vi "terminal_length_integrated.vi"(0 "ROI Ref":T3 {"Contours"."Type" items=["No Selection", "Point", "Line", "Rectangle", "Oval", "Polygon", "Free", "Annulus", "Unused2", "Unused3", "Broken Line", "Free Hand Line", "Rotated Rectangle"]}, 1 "Edge Options ROI Ref":T6={"Edge Polarity"=2, "Kernel Size"=5, "Width"=5, "Minimum Edge Strength"=50.0, "Interpolation Type"=enum."Zero Order", "Data Processing Method"=enum."Average"} {"Edge Polarity" items=["All Edges", "Rising Edges", "Falling Edges"]; "Minimum Edge Strength" format="%.2f"; "Width" step=2; "Kernel Size" step=2}, 2 "Search Direction ROI Ref":u32(ring)=3 items=["Left to Right", "Right to Left", "Top to Bottom", "Bottom to Top"], 3 "Line Options ROI Ref":T4={"Number of Lines"=1, "Type"=enum."First Edge Rake", "Min. Score"=10.0, "Max. Score"=1000.0, "Orientation"=0.0, "Angle Range"=30.0, "Angle Tolerance"=1.0, "Step Size"=5, "Min. SNR (db)"=0.0, "Min. Points (%)"=25.0, "Hough Iterations"=5} {"Min. Points (%)" min=0.0 max=100.0; "Min. SNR (db)" min=0.0; "Max. Score" min=0.0 max=1024.0; "Min. Score" min=0.0 max=1024.0 step=1.0}, 4 "ROI 1":T3 {"Contours"."Type" items=["No Selection", "Point", "Line", "Rectangle", "Oval", "Polygon", "Free", "Annulus", "Unused2", "Unused3", "Broken Line", "Free Hand Line", "Rotated Rectangle"]}, 5 "Edge Options ROI 1":T6={"Edge Polarity"=2, "Kernel Size"=5, "Width"=5, "Minimum Edge Strength"=50.0, "Interpolation Type"=enum."Zero Order", "Data Processing Method"=enum."Average"} {"Edge Polarity" items=["All Edges", "Rising Edges", "Falling Edges"]; "Minimum Edge Strength" format="%.2f"; "Width" step=2; "Kernel Size" step=2}, 6 "Search Direction ROI 1":u32(ring)=1 items=["Left to Right", "Right to Left", "Top to Bottom", "Bottom to Top"], 7 "error in (no error)":errorcluster, 8 "Image In":T8(plugin-control), 9 "Line Options ROI 1":T4={"Number of Lines"=1, "Type"=enum."First Edge Rake", "Min. Score"=10.0, "Max. Score"=1000.0, "Orientation"=0.0, "Angle Range"=30.0, "Angle Tolerance"=1.0, "Step Size"=5, "Min. SNR (db)"=0.0, "Min. Points (%)"=25.0, "Hough Iterations"=5} {"Min. Points (%)" min=0.0 max=100.0; "Min. SNR (db)" min=0.0; "Max. Score" min=0.0 max=1024.0; "Min. Score" min=0.0 max=1024.0 step=1.0}, 10 "Calibrated Image":T8, 11 "Edge Options ROI 2":T6={"Edge Polarity"=2, "Kernel Size"=5, "Width"=5, "Minimum Edge Strength"=50.0, "Interpolation Type"=enum."Zero Order", "Data Processing Method"=enum."Average"} {"Edge Polarity" items=["All Edges", "Rising Edges", "Falling Edges"]; "Minimum Edge Strength" format="%.2f"; "Width" step=2; "Kernel Size" step=2}, 12 "ROI 2":T3 {"Contours"."Type" items=["No Selection", "Point", "Line", "Rectangle", "Oval", "Polygon", "Free", "Annulus", "Unused2", "Unused3", "Broken Line", "Free Hand Line", "Rotated Rectangle"]}, 13 "Scan Direction ROI 2":u16(ring) items=["Left To Right", "Right To Left", "Top To Bottom", "Bottom To Top"], 14 "Process ROI 2":T2(ring), 15 "Step Size ROI 2":u32=5) -> (19 "overlay arrow lines":T1, 20 "Terminal Length":sgl, 27 "error out":errorcluster)   [LabVIEW 2019, in "Algorithm.lvclass"]
uses:
  FrameworkOverrides/Algorithm.lvclass
  <vilib>/vision/NI_Vision_Development_Module.lvlib
  <vilib>/vision/Image Controls.llb/IMAQ Image.ctl
  <vilib>/vision/Measure.llb/Edge Polarity.ctl
  <vilib>/vision/Measure.llb/Edge Options.ctl
  <vilib>/vision/Measure.llb/Straight Edge Process.ctl
  <vilib>/vision/Measure.llb/Straight Edge Options.ctl
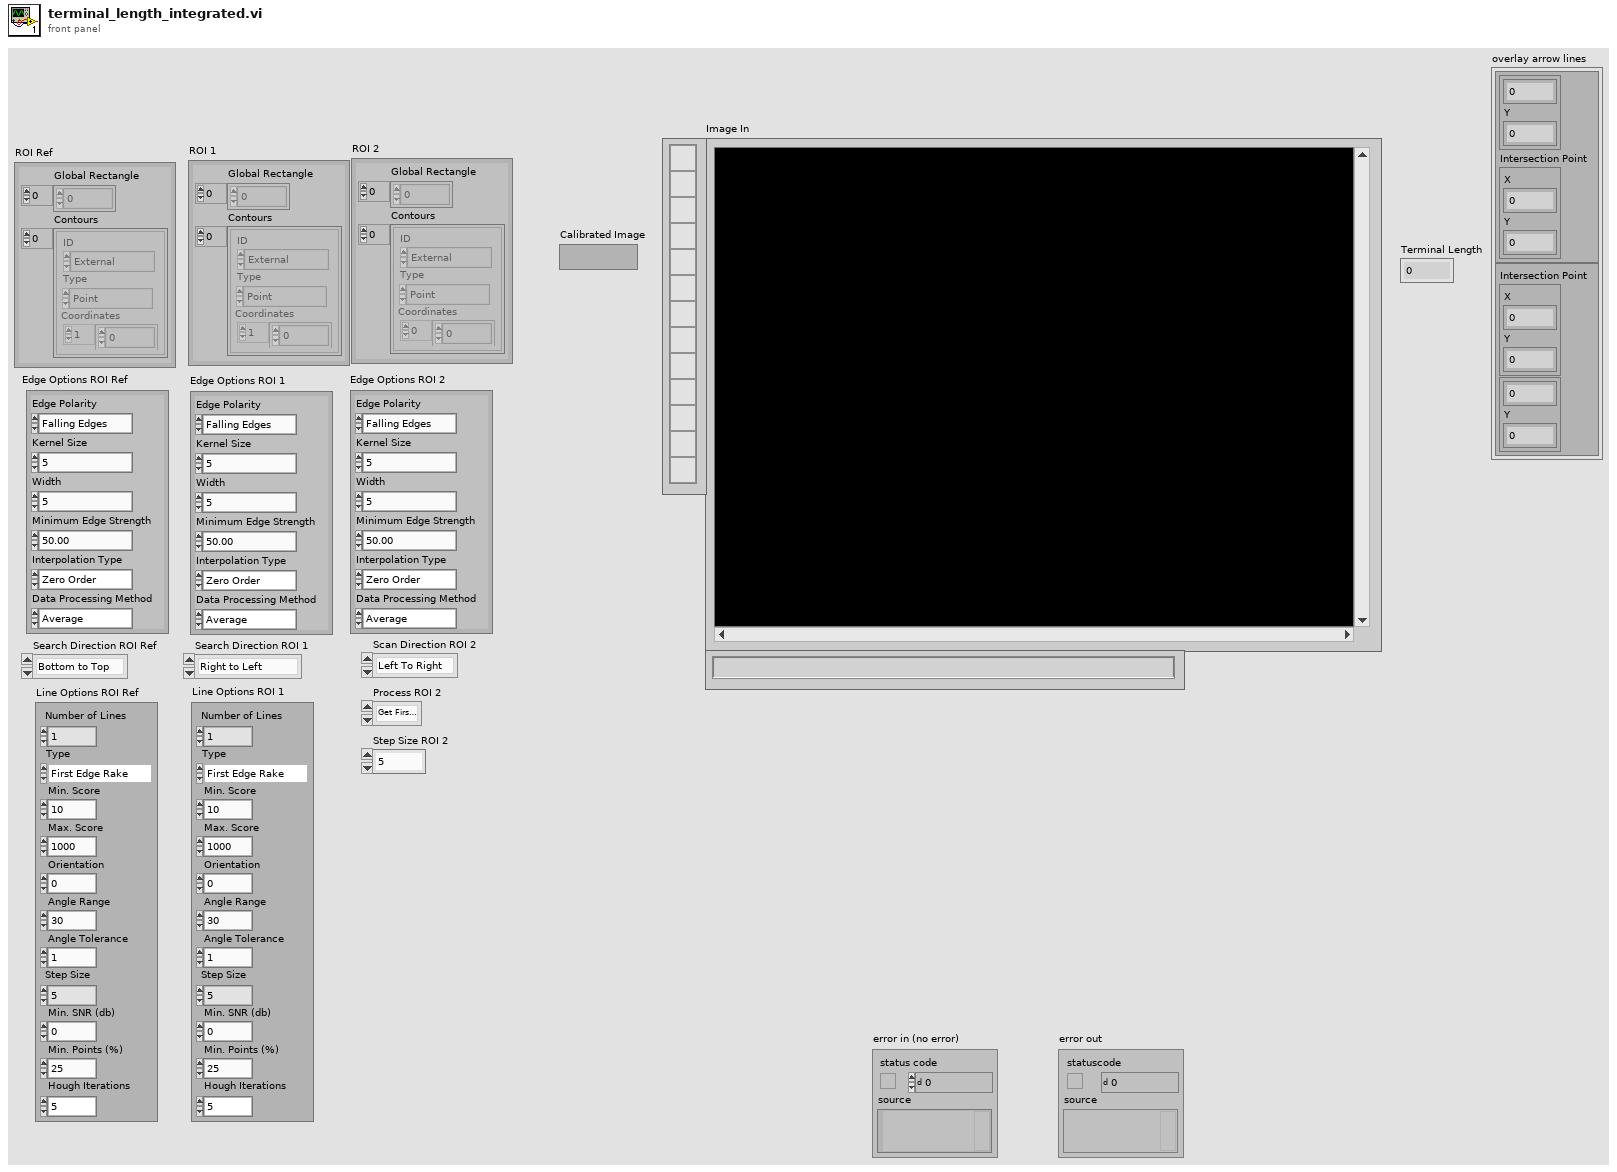
[diagram p1: front panel]
types:
  T1 = cluster{cluster{cluster{sgl, "Y":sgl}, "Intersection Point":cluster{"X":sgl, "Y":sgl}}, cluster{"Intersection Point":cluster{"X":sgl, "Y":sgl}, cluster{sgl, "Y":sgl}}}
  T2 = enum16{"Get First Edge", "Get First + Last Edge", "Get All Edges", "Get Best Edge"}
  T3 = cluster{"Global Rectangle":i32[], "Contours":cluster{"ID":enum32{"External", "Internal"}, "Type":u32, "Coordinates":i32[]}[]}
  T4 = typedef "Straight Edge Options.ctl" = cluster{"Number of Lines":i32, "Type":T5, "Min. Score":dbl, "Max. Score":dbl, "Orientation":dbl, "Angle Range":dbl, "Angle Tolerance":dbl, "Step Size":u32, "Min. SNR (db)":dbl, "Min. Points (%)":dbl, "Hough Iterations":i32}
  T5 = typedef "Straight Edge Process.ctl" = enum32{"First Edge Rake", "Best Edge Rake", "Hough Edge Rake", "First Edge Projection", "Best Edge Projection"}
  T6 = typedef "Edge Options.ctl" = cluster{"Edge Polarity":T7, "Kernel Size":u32, "Width":u32, "Minimum Edge Strength":sgl, "Interpolation Type":enum32{"Zero Order", "Bilinear", "Quadratic", "Cubic", "Bilinear Fixed"}, "Data Processing Method":enum32{"Average", "Median"}}
  T7 = typedef "Edge Polarity.ctl" = u32
  T8 = typedef "IMAQ Image.ctl" = refnum<image>
  T9 = cluster{"Point 1":cluster{"X":sgl, "Y":sgl}, "Point 2":cluster{"X":sgl, "Y":sgl}}
  T10 = cluster{"Point1 (Pixels)":cluster{"X":sgl, "Y":sgl}, "Point2 (Pixels)":cluster{"X":sgl, "Y":sgl}, "Point1 (Real-World)":cluster{"X":sgl, "Y":sgl}, "Point2 (Real-World)":cluster{"X":sgl, "Y":sgl}, "Angle (Pixel)":dbl, "Angle (Real-World)":dbl, "Score":dbl, "Straightness":dbl, "Average SNR (db)":dbl, "Calibration Valid":bool}[]
  T11 = cluster{"Point1 (Pixels)":cluster{"X":sgl, "Y":sgl}, "Point2 (Pixels)":cluster{"X":sgl, "Y":sgl}, "Point1 (Real-World)":cluster{"X":sgl, "Y":sgl}, "Point2 (Real-World)":cluster{"X":sgl, "Y":sgl}, "Angle (Pixel)":dbl, "Angle (Real-World)":dbl, "Score":dbl, "Straightness":dbl, "Average SNR (db)":dbl, "Calibration Valid":bool}
  T12 = typedef "Edge New.ctl" = cluster{"Location (Pixel)":cluster{"X":sgl, "Y":sgl}, "Location (Real-World)":cluster{"X":sgl, "Y":sgl}, "Distance (Pixel)":dbl, "Distance (Real-World)":dbl, "Strength":dbl, "Noise":dbl, "Rising?":bool}
  T13 = cluster{"Intersection Point":cluster{"X":sgl, "Y":sgl}, cluster{sgl, "Y":sgl}}
  T14 = cluster{cluster{sgl, "Y":sgl}, "Intersection Point":cluster{"X":sgl, "Y":sgl}}
  T15 = cluster{cluster{"Intersection Point":cluster{"X":sgl, "Y":sgl}, cluster{sgl, "Y":sgl}}, cluster{cluster{sgl, "Y":sgl}, "Intersection Point":cluster{"X":sgl, "Y":sgl}}}
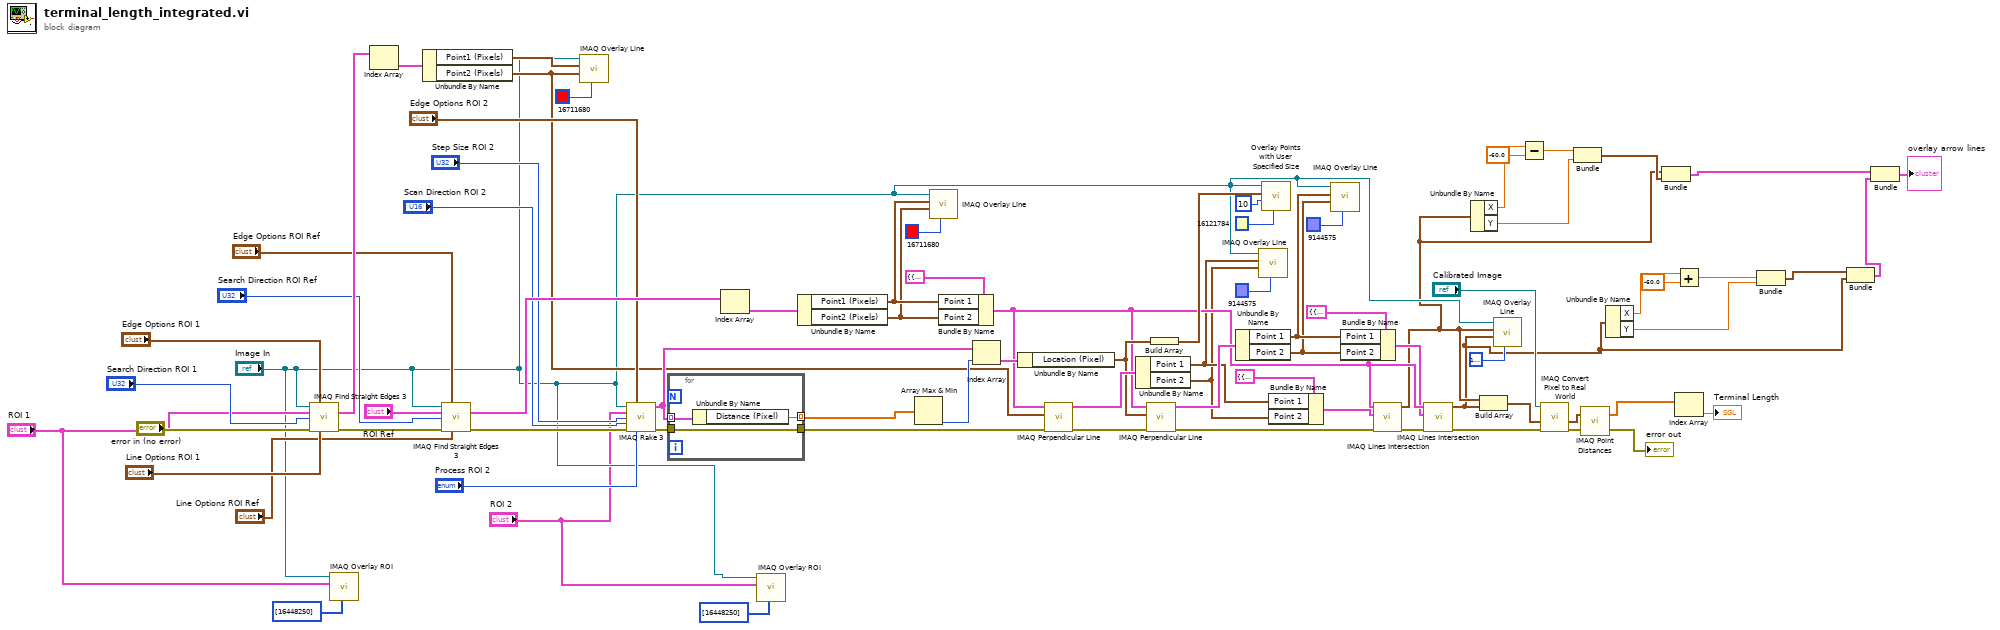
[diagram p0: block diagram]
diagram:
  n1 = call "IMAQ Find Straight Edges 3"("Image"="Image In", "Edge Options"="Edge Options ROI 1", "ROI Descriptor"="ROI 1", "Search Direction"="Search Direction ROI 1", "error in (no error)"="error in (no error)", "Line Options"="Line Options ROI 1") -> ("Straight Edges"=w77:T10, "error out"=w73:errorcluster)  [unwired: 5 in, 3 out]
  n2 = call "IMAQ Overlay ROI"("Colors (Green)"=u32[] [16448250], "ROI Descriptor"="ROI 1", "Image"="Image In") -> ()  [unwired: 7 in, 2 out]
  n3 = Index Array(array=w77) -> (element=w76:T11)  [unwired: 1 in]
  n4 = Unbundle By Name(w76) -> ("Point1 (Pixels)"=w75:cluster{"X":sgl, "Y":sgl}, "Point2 (Pixels)"=w50:cluster{"X":sgl, "Y":sgl})
  n5 = call "IMAQ Find Straight Edges 3"("Image"="Image In", "Edge Options"="Edge Options ROI Ref", "ROI Descriptor"="ROI Ref", "Search Direction"="Search Direction ROI Ref", "error in (no error)"=w73, "Line Options"="Line Options ROI Ref") -> ("Straight Edges"=w69:T10, "error out"=w66:errorcluster)  [unwired: 5 in, 3 out]
  n6 = call "IMAQ Overlay Line"("Color"=u32 16711680, "End Point"=w50, "Start Point"=w75, "Image"="Image In") -> ()  [unwired: 6 in, 2 out]
  n7 = call "IMAQ Rake 3"("Image"="Image In", "Edge Options"="Edge Options ROI 2", "ROI Descriptor"="ROI 2", "Step Size"="Step Size ROI 2", "Scan Direction"="Scan Direction ROI 2", "error in (no error)"=w66, "Process"="Process ROI 2") -> ("First Edges"=w59:T12[], "error out"=w61:errorcluster)  [unwired: 5 in, 2 out]
  n8 = for {
    tunnel: w61 -> [w81]
    tunnel: w59 -> [w83] mode=indexing
    tunnel: [w82] -> w60 mode=indexing
    tunnel: [w81] -> w34
    n9 = Unbundle By Name(w83) -> ("Distance (Pixel)"=w82:dbl)
  }
  n10 = Index Array(array=w69) -> (element=w68:T11)  [unwired: 1 in]
  n11 = call "IMAQ Overlay ROI"("Colors (Green)"=u32[] [16448250], "ROI Descriptor"="ROI 2", "Image"="Image In") -> ()  [unwired: 7 in, 2 out]
  n12 = Unbundle By Name(w68) -> ("Point1 (Pixels)"=w52:cluster{"X":sgl, "Y":sgl}, "Point2 (Pixels)"=w51:cluster{"X":sgl, "Y":sgl})
  n13 = Array Max & Min(array=w60) -> (min index (indices)=w54:i32)  [unwired: 3 out]
  n14 = call "IMAQ Overlay Line"("Color"=u32 16711680, "End Point"=w51, "Start Point"=w52, "Image"="Image In") -> ()  [unwired: 6 in, 2 out]
  n15 = Bundle By Name(cluster=T9 {"Point 1"={"X"=0.0, "Y"=0.0}, "Point 2"={"X"=0.0, "Y"=0.0}} ("Line"), "Point 1"=w52, "Point 2"=w51) -> (w44:T9)
  n16 = Index Array(array=w59, index=w54) -> (element=w58:T12)
  n17 = Unbundle By Name(w58) -> ("Location (Pixel)"=w47:cluster{"X":sgl, "Y":sgl})
  n18 = call "IMAQ Perpendicular Line"("error in (no error)"=w34, "Point"=w50, "Line"=w44) -> ("error out"=w33:errorcluster, "Perpendicular Line"=w49:T9)  [unwired: 6 in, 1 out]
  n19 = Unbundle By Name(w49) -> ("Point 1"=w41:cluster{"X":sgl, "Y":sgl}, "Point 2"=w40:cluster{"X":sgl, "Y":sgl})
  n20 = call "IMAQ Perpendicular Line"("error in (no error)"=w33, "Point"=w47, "Line"=w44) -> ("error out"=w32:errorcluster, "Perpendicular Line"=w45:T9)  [unwired: 6 in, 1 out]
  n21 = Build Array(w47) -> (w57:cluster{"X":sgl, "Y":sgl}[])
  n22 = Unbundle By Name(w45) -> ("Point 1"=w38:cluster{"X":sgl, "Y":sgl}, "Point 2"=w37:cluster{"X":sgl, "Y":sgl})
  n23 = call "IMAQ Overlay Line"("Color"=u32 9144575, "End Point"=w40, "Start Point"=w41, "Image"="Image In") -> ()  [unwired: 6 in, 2 out]
  n24 = call "Overlay Points with User Specified Size.vi"("Color"=u32 16121784, "Point Diameter (5)"=u32 10, "Points"=w57, "Image In"="Image In") -> ()  [unwired: 6 in, 2 out]
  n25 = Bundle By Name(cluster=T9 {"Point 1"={"X"=0.0, "Y"=0.0}, "Point 2"={"X"=0.0, "Y"=0.0}} ("Line 2"), "Point 1"=w41, "Point 2"=w40) -> (w39:T9)
  n26 = call "IMAQ Overlay Line"("Color"=u32 9144575, "End Point"=w37, "Start Point"=w38, "Image"="Image In") -> ()  [unwired: 6 in, 2 out]
  n27 = Bundle By Name(cluster=T9 {"Point 1"={"X"=0.0, "Y"=0.0}, "Point 2"={"X"=0.0, "Y"=0.0}} ("Line 2"), "Point 1"=w38, "Point 2"=w37) -> (w36:T9)
  n28 = call "IMAQ Lines Intersection"("error in (no error)"=w32, "Line 2"=w39, "Line 1"=w44) -> ("error out"=w31:errorcluster, "Intersection Point"=w3:cluster{"X":sgl, "Y":sgl})  [unwired: 6 in, 1 out]
  n29 = call "IMAQ Lines Intersection"("error in (no error)"=w31, "Line 2"=w36, "Line 1"=w44) -> ("error out"=w30:errorcluster, "Intersection Point"=w1:cluster{"X":sgl, "Y":sgl})  [unwired: 6 in, 1 out]
  n30 = Unbundle By Name(w3) -> ("X"=w15:sgl, "Y"=w12:sgl)
  n31 = Build Array(w3, w1) -> (w29:cluster{"X":sgl, "Y":sgl}[])
  n32 = call "IMAQ Overlay Line"("Color"=u32 16777226, "End Point"=w1, "Start Point"=w3, "Image"="Image In") -> ()  [unwired: 6 in, 2 out]
  n33 = Subtract(x=w15, y=sgl -60.0) -> (x-y=w13:sgl)
  n34 = call "IMAQ Convert Pixel to Real World"("error in (no error)"=w30, "Array of Pixel Coordinates"=w29, "Calibrated Image"="Calibrated Image") -> ("error out"=w24:errorcluster, "Array of Real World Coordinates"=w28:cluster{"X":sgl, "Y":sgl}[])  [unwired: 3 in, 4 out]
  n35 = Bundle(w13, "Y"=w12) -> (w4:cluster{sgl, "Y":sgl})  [unwired: 1 in]
  n36 = call "IMAQ Point Distances"("Points"=w28, "error in (no error)"=w24) -> ("Distances"=w27:sgl[], "error out"=→"error out":errorcluster)  [unwired: 3 in]
  n37 = Unbundle By Name(w1) -> ("X"=w11:sgl, "Y"=w9:sgl)
  n38 = Bundle("Intersection Point"=w3, w4) -> (w7:T13)  [unwired: 1 in]
  n39 = Add(x=w11, y=sgl -60.0) -> (x+y=w8:sgl)
  n40 = Index Array(array=w27) -> (element=→"Terminal Length":sgl)  [unwired: 1 in]
  n41 = Bundle(w8, "Y"=w9) -> (w2:cluster{sgl, "Y":sgl})  [unwired: 1 in]
  n42 = Bundle(w2, "Intersection Point"=w1) -> (w6:T14)  [unwired: 1 in]
  n43 = Bundle(w7, w6) -> (→"overlay arrow lines":T15)  [unwired: 1 in]
